vi "Open.vi"(8 "error in (no error)":errorcluster caption="entrée d'erreur (pas d'erreur)", 11 "Class Relay_Board 16_Relay_CH340 en entrée":refnum<class "Class Relay_Board 16_Relay_Acer_Micro.lvclass">) -> (0 "error out":errorcluster caption="sortie d'erreur", 3 "Class Relay_Board 16_Relay_CH340 en sortie":refnum<class "Class Relay_Board 16_Relay_Acer_Micro.lvclass">)   [LabVIEW 2020, in "Library Instrument & Equipement.lvlib" / "Library Relay_Board.lvlib" / "Class Relay_Board 16_Relay_Acer_Micro.lvclass"]
uses:
  Class Relay_Board 16_Relay_Acer_Micro.lvclass
  C:/Users/ngarcin/OneDrive - Altyor/Standard TB/Class/Relay_Board/Relay_Board (Default)/Class Relay_Board (Default).lvclass
  Class Relay_Board 16_Relay_Acer_Micro.lvclass/Class Relay_Board 16_Relay_Acer_Micro.ctl
  <vilib>/Instr/_visa.llb/VISA Configure Serial Port (Instr).vi
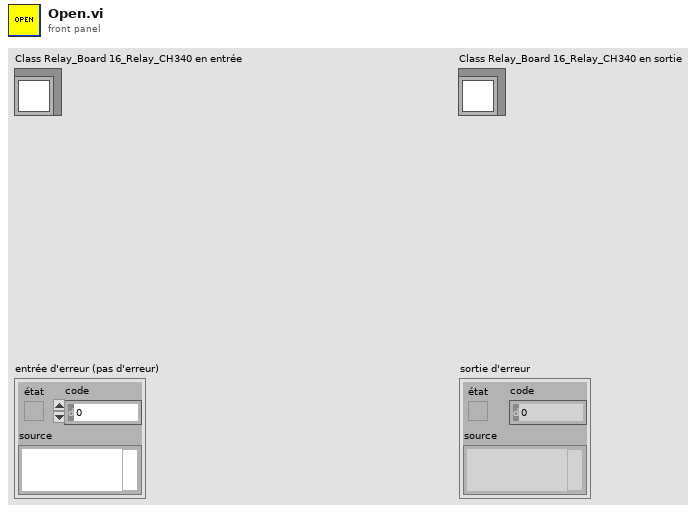
[diagram p1: front panel]
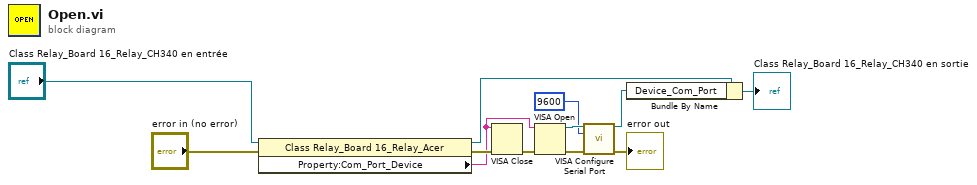
[diagram p0: block diagram]
diagram:
  n1 = property class="Class Relay_Board 16_Relay_Acer"(reference="Class Relay_Board 16_Relay_CH340 en entrée", error in="error in (no error)") -> (reference out=w4:refnum<class "Class Relay_Board 16_Relay_Acer_Micro.lvclass">, error out=w6:errorcluster, "Property:Com_Port_Device"=w5:string)
  n2 = VISA Close(VISA resource name=w5, error in (no error)=w6) -> (error out=w8:errorcluster)
  n3 = VISA Open(error in (no error)=w8, VISA resource name=w5) -> (VISA resource name=w12:refnum<visa-resource-name>, error out=w10:errorcluster)  [unwired: 3 in]
  n4 = call-poly "VISA Configure Serial Port"("VISA resource name"=w12, "baud rate (9600)"=u32 9600, "error in (no error)"=w10) -> ("VISA resource name out"=w1:refnum<visa-resource-name>, "error out"=→"error out":errorcluster)  [unwired: 11 in]
  n5 = Bundle By Name(cluster=w4, "Device_Com_Port"=w1) -> (→"Class Relay_Board 16_Relay_CH340 en sortie":refnum<class "Class Relay_Board 16_Relay_Acer_Micro.lvclass">)
